vi "ConvertToMessages.vi"(8 "error in (no error)":errorcluster, 11 "ServiceDefs":T5[](array[typedef])) -> (0 "error out":errorcluster, 3 "Messages":T1[](array[typedef]))   [LabVIEW 2017, in "MessageGen.lvlib"]
uses:
  <vilib>/addons/InsightCM/MessageBus/CodeGen/MessageGen.lvlib
  <vilib>/addons/InsightCM/MessageBus/CodeGen/controls/ServiceDef.ctl
  <vilib>/addons/InsightCM/MessageBus/CodeGen/controls/MessageDef.ctl
  <vilib>/addons/InsightCM/MessageBus/CodeGen/controls/ParameterDef.ctl
  <vilib>/addons/InsightCM/MessageBus/CodeGen/controls/MessageData.ctl
  <vilib>/addons/InsightCM/MessageBus/CodeGen/controls/MessageType.ctl
  <vilib>/addons/InsightCM/MessageBus/CodeGen/controls/Parameter.ctl
  <vilib>/addons/InsightCM/MessageBus/CodeGen/controls/ParameterType.ctl
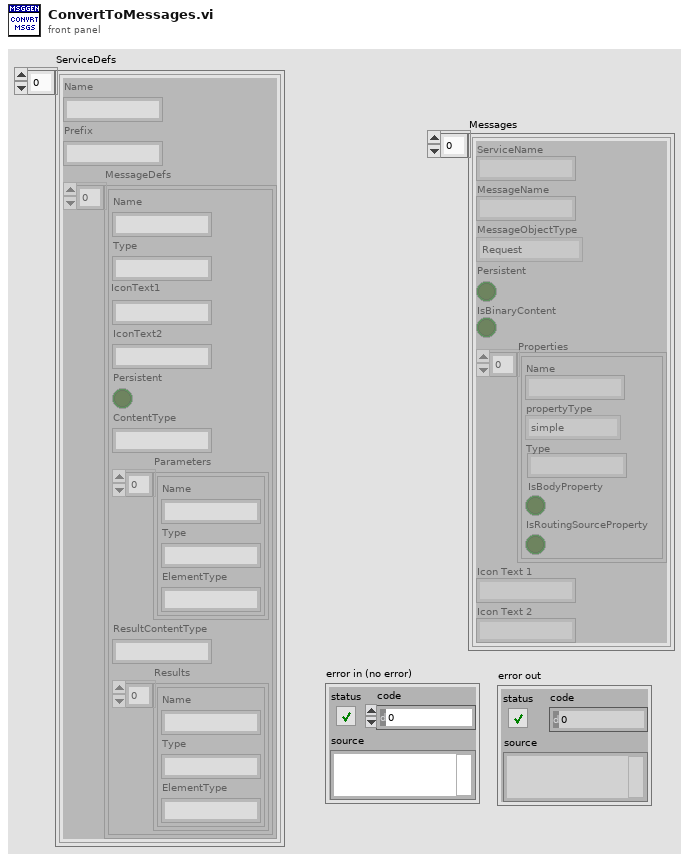
[diagram p1: front panel]
types:
  T1 = typedef "MessageGen.lvlib/MessageData.ctl" = cluster{"ServiceName":string, "MessageName":string, "MessageObjectType":T2, "Persistent":bool, "IsBinaryContent":bool, "Properties":T3[], "Icon Text 1":string, "Icon Text 2":string}
  T2 = typedef "MessageGen.lvlib/MessageType.ctl" = enum16{"Request", "Response", "Broadcast", "RoutedMessage"}
  T3 = typedef "MessageGen.lvlib/Parameter.ctl" = cluster{"Name":string, "propertyType":T4, "Type":string, "IsBodyProperty":bool, "IsRoutingSourceProperty":bool}
  T4 = typedef "MessageGen.lvlib/ParameterType.ctl" = enum16{"simple", "bytearray", "dateTime", "list", "map", "object"}
  T5 = typedef "MessageGen.lvlib/ServiceDef.ctl" = cluster{"Name":string, "Prefix":string, "MessageDefs":T6[]}
  T6 = typedef "MessageGen.lvlib/MessageDef.ctl" = cluster{"Name":string, "Type":string, "IconText1":string, "IconText2":string, "Persistent":bool, "ContentType":string, "Parameters":T7[], "ResultContentType":string, "Results":T7[]}
  T7 = typedef "MessageGen.lvlib/ParameterDef.ctl" = cluster{"Name":string, "Type":string, "ElementType":string}
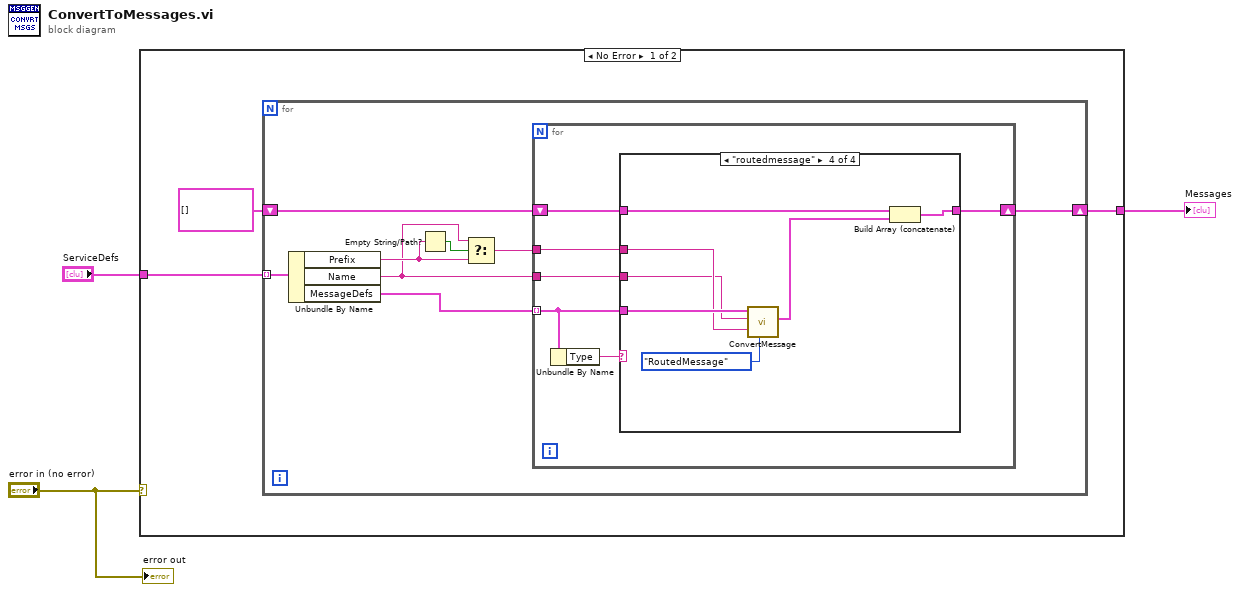
[diagram p0: block diagram]
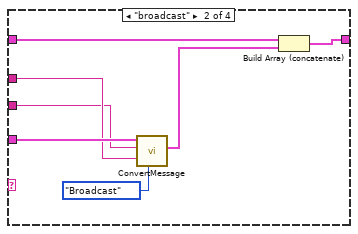
[diagram p3: hidden frame]
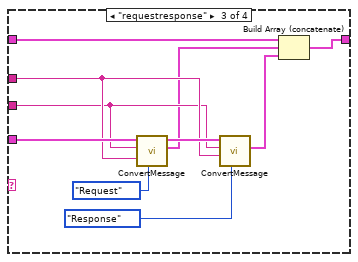
[diagram p4: hidden frame]
diagram:
  n1 = case shown="No Error" "error in (no error)" {
    tunnel: "ServiceDefs" -> [w6 _]
    tunnel: [w5 _] -> w2
    frame No Error {
      n2 = for {
        tunnel: w6 -> [w14] mode=indexing
        shift-right: [w7] -> w5
        shift-left: T1[] [] -> [w9]
        n3 = Unbundle By Name(w14) -> ("Prefix"=w11:string, "Name"=w8:string, "MessageDefs"=w13:T6[])
        n4 = Empty String/Path?(string/path=w11) -> (empty?=w12:bool)
        n5 = Select(t=w8, s=w12, f=w11) -> (s? t:f=w10:string)
        n6 = for {
          tunnel: w13 -> [w18] mode=indexing
          tunnel: w10 -> [w17]
          shift-right: [w15] -> w7
          shift-left: w9 -> [w16]
          tunnel: w8 -> [w19]
          n7 = Unbundle By Name(w18) -> ("Type"=w20:string)
          n8 = case shown="\"routedmessage\"" w20 {
            tunnel: w19 -> [_ w26 w35 w43]
            tunnel: w18 -> [_ w28 w38 w45]
            tunnel: w17 -> [_ w27 w36 w44]
            tunnel: w16 -> [w21 w24 w32 w41]
            tunnel: [w21 w22 w30 w39] -> w15
            frame Default {
            }
            frame "broadcast" {
              n9 = call <vilib>:"ConvertMessage.vi"("MessageObjectType"=MessageType."Broadcast", "ServicePrefix"=w27, "ServiceName"=w26, "MessageDef in"=w28) -> ("Message"=w23:T1)  [unwired: 6 in, 1 out]
              n10 = Build Array (concatenate)(w24, w23) -> (w22:T1[])
            }
            frame "requestresponse" {
              n11 = call <vilib>:"ConvertMessage.vi"("MessageObjectType"=MessageType."Request", "ServicePrefix"=w36, "ServiceName"=w35, "MessageDef in"=w38) -> ("Message"=w31:T1, "MessageDef out"=w37:T6)  [unwired: 6 in]
              n12 = call <vilib>:"ConvertMessage.vi"("MessageObjectType"=MessageType."Response", "ServicePrefix"=w36, "ServiceName"=w35, "MessageDef in"=w37) -> ("Message"=w29:T1)  [unwired: 6 in, 1 out]
              n13 = Build Array (concatenate)(w32, w31, w29) -> (w30:T1[])
            }
            frame "routedmessage" {
              n14 = call <vilib>:"ConvertMessage.vi"("MessageObjectType"=MessageType."RoutedMessage", "ServicePrefix"=w44, "ServiceName"=w43, "MessageDef in"=w45) -> ("Message"=w40:T1)  [unwired: 6 in, 1 out]
              n15 = Build Array (concatenate)(w41, w40) -> (w39:T1[])
            }
          }
        }
      }
    }
    frame Error {
    }
  }
  "Messages" <- w2
  "error out" <- "error in (no error)"
